vi "Open.vi"(8 "error in (no error)":errorcluster, 11 "NI Digital in":refnum<class "No Output.lvclass">) -> (0 "error out":errorcluster, 3 "NI Digital out":refnum<class "No Output.lvclass">)   [LabVIEW 2024, in "No Output.lvclass"]
doc: "No Output.lvclass:Open.vi\n\nThis is the Open VI for the No Output class.\n\nInstrument Communication Module Version 1.0\nOctober, 2020 Original Code Consulting Davita Bird\n www.originalcode.com"
uses:
  No Output.lvclass
  No Output.lvclass/No Output.ctl
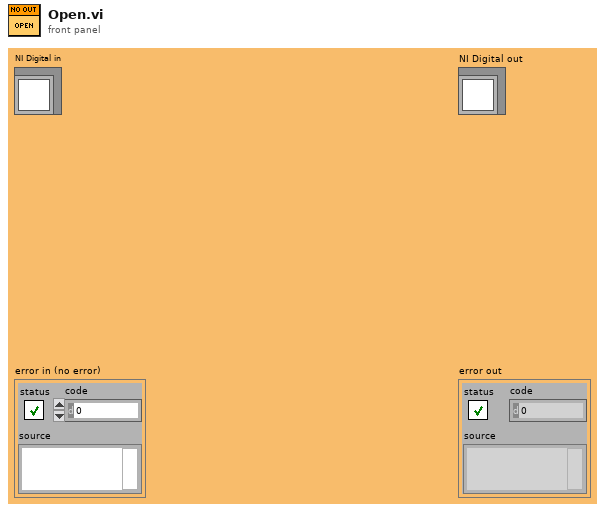
[diagram p1: front panel]
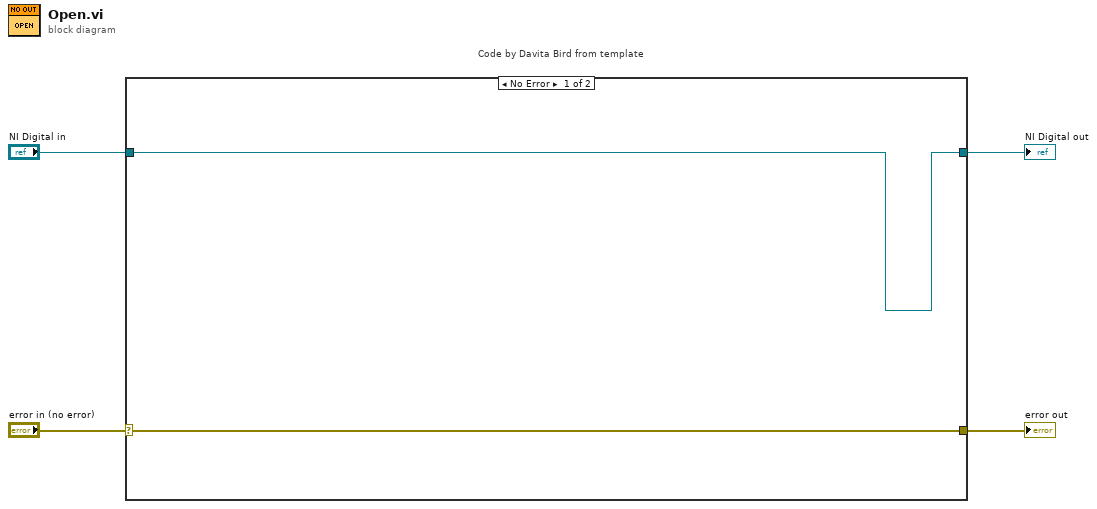
[diagram p0: block diagram]
diagram:
  n1 = case "Code by Davita Bird from template" shown="No Error" "error in (no error)" {
    selector: "error in (no error)" -> [w5 w8]
    tunnel: [w5 w8] -> w3
    tunnel: [w6 w7] -> w2
    tunnel: "NI Digital in" -> [w6 w7]
    frame No Error {
    }
    frame Error {
    }
  }
  "error out" <- w3
  "NI Digital out" <- w2
